vi "KM101_CreatActiveX.vi"() -> (1 "KIM引用":refnum<k7>)   [LabVIEW 2018, in "KIM101lib.lvlib"]
uses:
  KIM101lib.lvlib
  <vilib>/Utility/error.llb/DialogType.ctl
panel:
  in  "APTPZMotor":refnum<k7>(container)
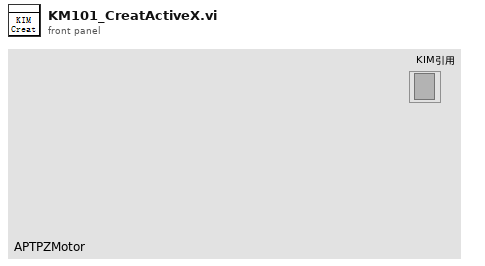
[diagram p1: front panel]
types:
  T1 = typedef "DialogType.ctl" = u16
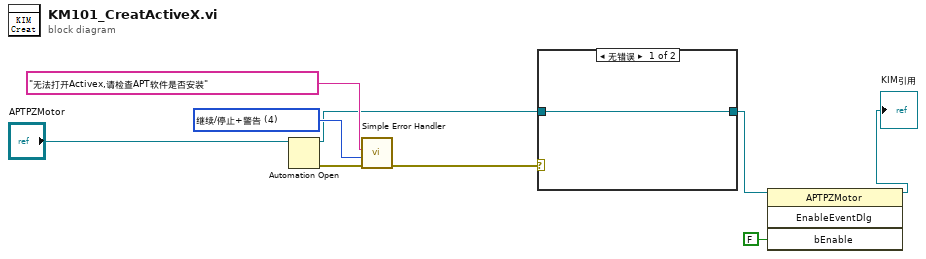
[diagram p0: block diagram]
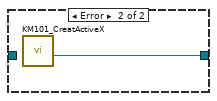
[diagram p2: hidden frame]
diagram:
  w7 = T1 4 items=["无对话框", "确定信息", "继续或停止信息", "确定信息＋警告", "继续/停止+警告"] ("type of dialog (OK msg:1)")
  n1 = Automation Open(Automation Refnum="APTPZMotor") -> (Automation Refnum=w4:refnum<k7>, error out=w8:errorcluster)  [unwired: 3 in]
  n2 = call <vilib>:"Simple Error Handler.vi"("error source (\" \")"="无法打开Activex,请检查APT软件是否安装" ("error source (\" \")"), "type of dialog (OK msg:1)"=w7, "error in (no error)"=w8) -> ("error out"=w6:errorcluster)  [unwired: 2 in, 4 out]
  n3 = case shown="无错误" w6 {
    tunnel: [w10 w11] -> w3
    tunnel: w4 -> [w10 _]
    frame No Error {
    }
    frame Error {
      n4 = call "KM101_CreatActiveX.vi"() -> ("KIM引用"=w11:refnum<k7>)  [unwired: 11 in]
    }
  }
  n5 = invoke class="APTPZMotor" method="EnableEventDlg"(reference=w3, "bEnable"=FALSE) -> (reference out=→"KIM引用":refnum<k7>)  [unwired: 2 in, 3 out]
